vi "Read Time Stamp.vi"(8 "error in (no error)":errorcluster, 11 "time in":refnum<class "Timestamp.lvclass">) -> (0 "error out":errorcluster, 2 "Time Stamp":timestamp, 3 "time out":refnum<class "Timestamp.lvclass">)   [LabVIEW 2020, in "Example Source.lvlib" / "Timestamp.lvclass"]
uses:
  Timestamp.lvclass
  Timestamp.lvclass/Timestamp.ctl
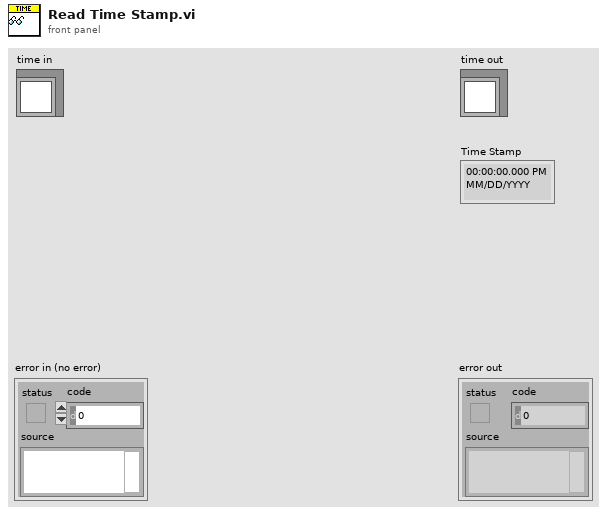
[diagram p1: front panel]
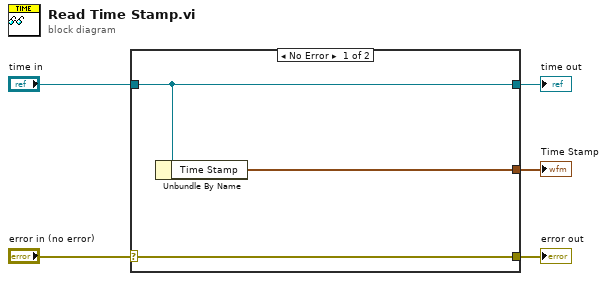
[diagram p0: block diagram]
diagram:
  n1 = case shown="No Error" "error in (no error)" {
    selector: "error in (no error)" -> [w8 w9]
    tunnel: [w8 w9] -> w4
    tunnel: [w7 w10] -> w2
    tunnel: "time in" -> [w7 w10]
    tunnel: [w6 _] -> w1
    frame No Error {
      n2 = Unbundle By Name(w7) -> ("Time Stamp"=w6:timestamp)
    }
    frame Error {
    }
  }
  "error out" <- w4
  "time out" <- w2
  "Time Stamp" <- w1
